vi "Drive Immediate.vi"(7 "Description":string, 8 "Command Info In":T1, 9 "Deadband Value":dbl=0.01, 10 "Right Setpoint":dbl, 11 "Left Setpoint":dbl) -> (0 "Command Info Out":T1)   [LabVIEW 2017]
doc: "Often used for joystick control, this VI checks to see that the joystick axes are outside the deadband and updates the motors appropriately."
uses:
  <vilib>/Rock Robotics/WPI/Framework/Command Status Info.ctl
  <vilib>/Rock Robotics/WPI/Framework/Completion Status.ctl
  <vilib>/Rock Robotics/WPI/Framework/Completion Notifier.ctl
  Implementation/Drive Setpoints.ctl
  Implementation/Drive Operations.ctl
panel:
  in  "Right Setpoint":dbl
  in  "Description":string
  out "Command Info Out":T1
  in  "Command Info In":T1
  in  "Left Setpoint":dbl
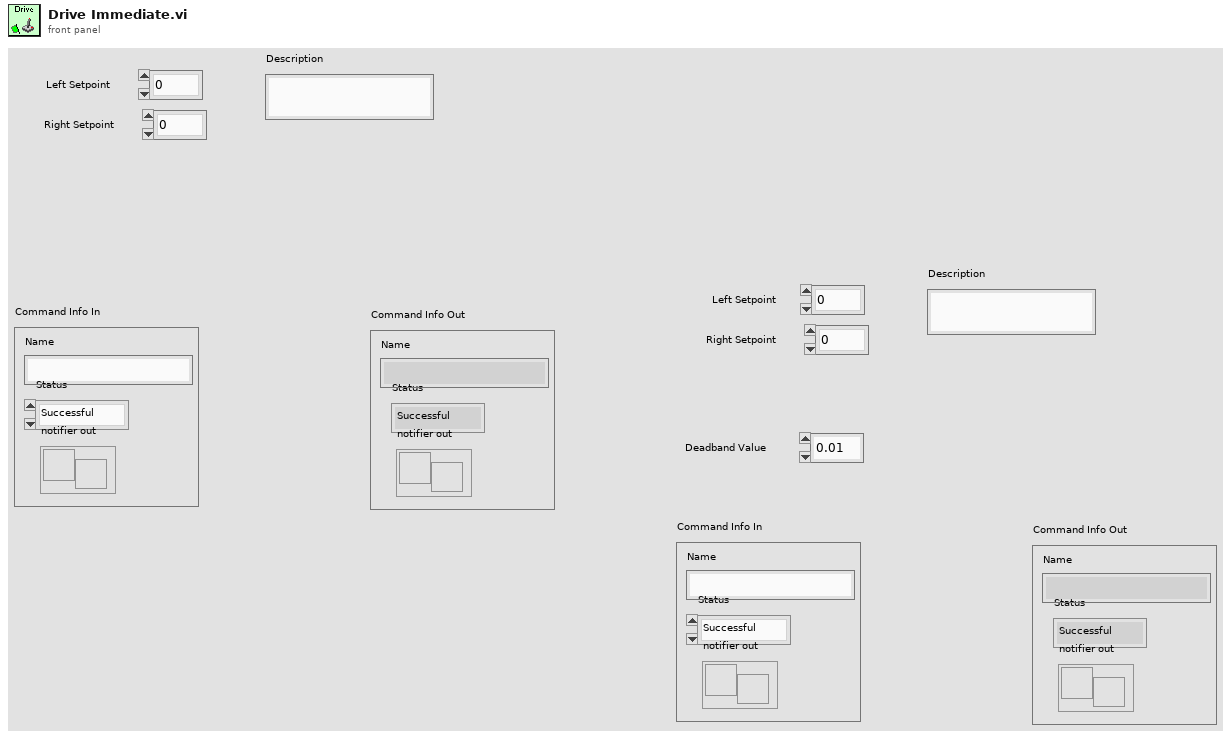
[diagram p1: front panel]
types:
  T1 = typedef "Command Status Info.ctl" = cluster{"Name":string, "Status":T2, "notifier out":T3}
  T2 = typedef "Completion Status.ctl" = enum16{"Successful", "Aborted", "Incomplete"}
  T3 = typedef "Completion Notifier.ctl" = refnum<notifier>
  T4 = typedef "Drive Setpoints.ctl" = cluster{"Operation":T5, "Left Setpoint":dbl, "Right Setpoint":dbl, "Duration":dbl}
  T5 = typedef "Drive Operations.ctl" = enum16{"Reserve", "Read Current", "Immediate", "Drive for Time", "Drive for Distance"}
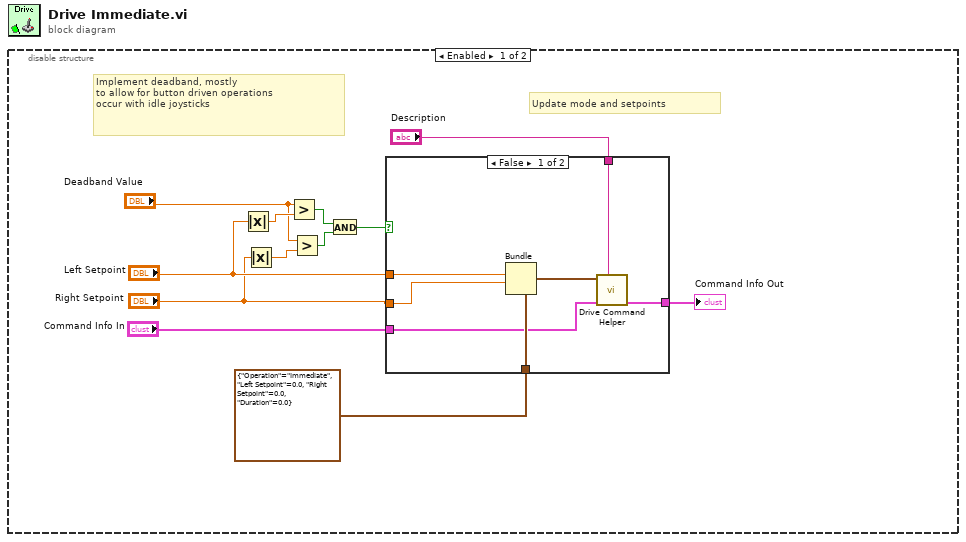
[diagram p0: block diagram]
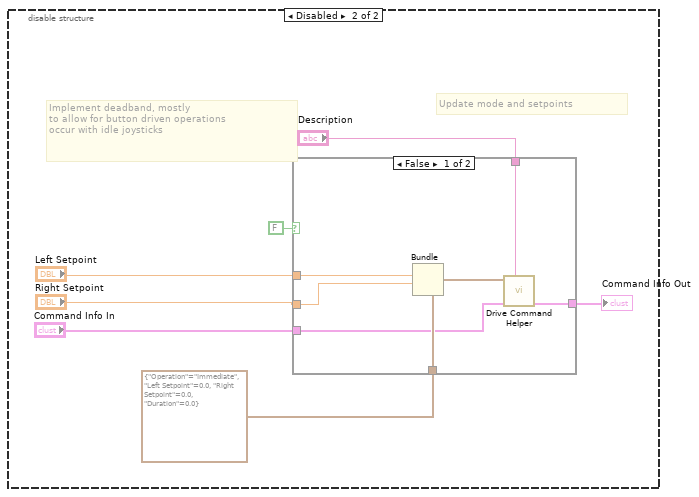
[diagram p3: hidden frame]
diagram:
  n1 = disable-structure shown="Enabled" {
    frame Enabled {
      # "Implement deadband, mostly\nto allow for button driven operations\noccur with idle joysticks"
      # "Update mode and setpoints"
      n2 = Absolute Value(x="Left Setpoint") -> (abs(x)=w12:dbl)
      n3 = Absolute Value(x="Right Setpoint") -> (abs(x)=w4:dbl)
      n4 = Greater?(x="Deadband Value", y=w12) -> (0:w6:bool)
      n5 = Greater?(x="Deadband Value", y=w4) -> (0:w2:bool)
      n6 = And(x=w6, y=w2) -> (x .and. y?=w5:bool)
      n7 = case shown="False" w5 {
        tunnel: "Left Setpoint" -> [w19 _]
        tunnel: T4 {"Operation"=enum."Immediate", "Left Setpoint"=0.0, "Right Setpoint"=0.0, "Duration"=0.0} ("SubSystem Data") -> [w18 _]
        tunnel: [w17 w20] -> w11
        tunnel: "Command Info In" -> [w16 w20]
        tunnel: "Description" -> [w14 _]
        tunnel: "Right Setpoint" -> [w13 _]
        frame False {
          n8 = Bundle(cluster=w18, "Left Setpoint"=w19, "Right Setpoint"=w13) -> (w15:T4)  [unwired: 2 in]
          n9 = call "Drive Command Helper.vi"("Description"=w14, "Command Info In"=w16, "SubSystem Data"=w15) -> ("Command Info Out"=w17:T1)  [unwired: 6 in, 2 out]
        }
        frame True {
        }
      }
      "Command Info Out" <- w11
    }
    frame Disabled {
      # "Implement deadband, mostly\nto allow for button driven operations\noccur with idle joysticks"
      # "Update mode and setpoints"
      n10 = case shown="False" FALSE {
        tunnel: "Left Setpoint" -> [w34 _]
        tunnel: T4 {"Operation"=enum."Immediate", "Left Setpoint"=0.0, "Right Setpoint"=0.0, "Duration"=0.0} ("SubSystem Data") -> [w33 _]
        tunnel: [w32 w35] -> w27
        tunnel: "Command Info In" -> [w31 w35]
        tunnel: "Description" -> [w29 _]
        tunnel: "Right Setpoint" -> [w28 _]
        frame False {
          n11 = Bundle(cluster=w33, "Left Setpoint"=w34, "Right Setpoint"=w28) -> (w30:T4)  [unwired: 2 in]
          n12 = call "Drive Command Helper.vi"("Description"=w29, "Command Info In"=w31, "SubSystem Data"=w30) -> ("Command Info Out"=w32:T1)  [unwired: 6 in, 2 out]
        }
        frame True {
        }
      }
      "Command Info Out" <- w27
    }
  }
